vi "Keithley 2420 avg resistance.vi"() -> ()   [LabVIEW 2013]
uses:
  <instrlib>/Keithley 24XX/Public/Data/Read (Single Point).vi
  <instrlib>/Keithley 24XX/Keithley 24XX.lvlib
panel:
  in  "stop":bool
  out "Waveform Chart":cluster{sgl, sgl}(graph)
  out "avg resistance (kOhm)":sgl
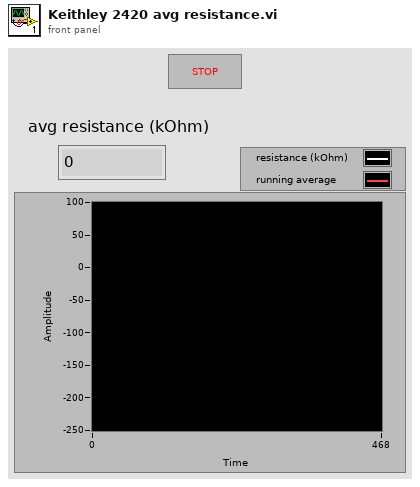
[diagram p1: front panel]
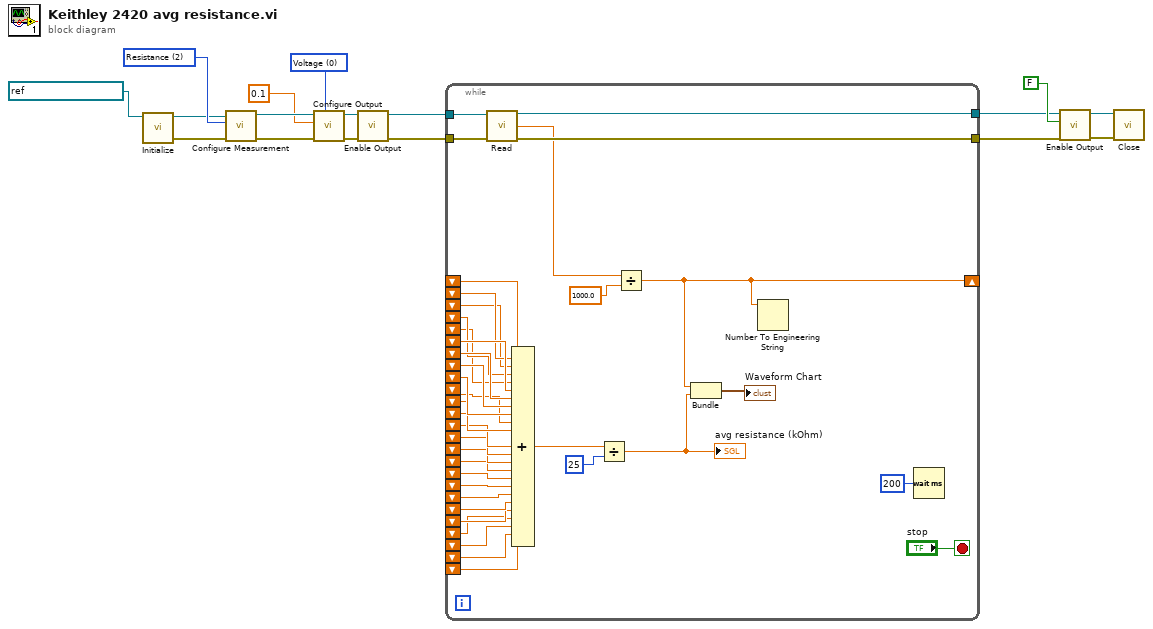
[diagram p0: block diagram]
diagram:
  w11 = u16 0 items=["Voltage", "Current"] ("Source Mode  (0: Voltage)")
  w16 = u16 2 items=["Volts", "Current", "Resistance"] ("Function (0: Volts)")
  n1 = call <instrlib>:"Initialize.vi"("VISA resource name"=refnum<visa-resource-name> "GPIB1::24::INSTR") -> ("error out"=w8:errorcluster, "VISA resource name out"=w9:refnum<visa-resource-name>)  [unwired: 9 in]
  n2 = call <instrlib>:"Configure Measurement.vi"("error in (no error)"=w8, "Function (0: Volts)"=w16, "VISA resource name"=w9) -> ("error out"=w15:errorcluster, "VISA resource name out"=w14:refnum<visa-resource-name>)  [unwired: 7 in]
  n3 = call <instrlib>:"Configure Output.vi"("Source Mode  (0: Voltage)"=w11, "error in (no error)"=w15, "Output Level (0)"=0.1, "VISA resource name"=w14) -> ("error out"=w13:errorcluster, "VISA resource name out"=w12:refnum<visa-resource-name>)  [unwired: 6 in]
  n4 = call <instrlib>:"Enable Output.vi"("error in (no error)"=w13, "VISA resource name"=w12) -> ("error out"=w1:errorcluster, "VISA resource name out"=w2:refnum<visa-resource-name>)  [unwired: 8 in]
  n5 = while {
    tunnel: [w54] -> w4
    tunnel: [w53] -> w3
    tunnel: w2 -> [w52]
    tunnel: w1 -> [w51]
    shift-right: [w24] -> _
    shift-left: _ -> [w50]
    shift-left: _ -> [w49]
    shift-left: _ -> [w48]
    shift-left: _ -> [w47]
    shift-left: _ -> [w46]
    shift-left: _ -> [w45]
    shift-left: _ -> [w44]
    shift-left: _ -> [w43]
    shift-left: _ -> [w42]
    shift-left: _ -> [w41]
    shift-left: _ -> [w35]
    shift-left: _ -> [w31]
    shift-left: _ -> [w32]
    shift-left: _ -> [w33]
    shift-left: _ -> [w34]
    shift-left: _ -> [w29]
    shift-left: _ -> [w28]
    shift-left: _ -> [w27]
    shift-left: _ -> [w26]
    shift-left: _ -> [w25]
    shift-left: _ -> [w19]
    shift-left: _ -> [w20]
    shift-left: _ -> [w21]
    shift-left: _ -> [w22]
    shift-left: _ -> [w23]
    stop <- "stop" stop-if-true
    n6 = call-poly <instrlib>:"Read.vi"("VISA resource name"=w52, "error in (no error)"=w51) -> ("VISA resource name out"=w54:refnum<visa-resource-name>, "Resistance"=w37:sgl, "error out"=w53:errorcluster)  [unwired: 7 in, 4 out]
    n7 = Compound Arithmetic op=ADD(w23, w22, w21, w20, w19, w50, w49, w48, w47, w46, w45, w44, w43, w42, w41, w35, w31, w32, w33, w34, w29, w28, w27, w26, w25) -> (w40:sgl)
    n8 = Divide(x=w40, y=25 ("# of measurements to average")) -> (x/y=w39:sgl)
    "avg resistance (kOhm)" <- w39
    n9 = Divide(x=w37, y=sgl 1000.0) -> (x/y=w24:sgl)
    n10 = Bundle(w24, w39) -> (→"Waveform Chart":cluster{sgl, sgl})  [unwired: 1 in]
    n11 = Number To Engineering String(4:w24) -> ()  [unwired: 3 in, 1 out]
    n12 = Wait (ms)(milliseconds to wait=u32 200) -> ()  [unwired: 1 out]
  }
  n13 = call <instrlib>:"Enable Output.vi"("error in (no error)"=w3, "Enable Output (T: Enable)"=FALSE, "VISA resource name"=w4) -> ("error out"=w5:errorcluster, "VISA resource name out"=w7:refnum<visa-resource-name>)  [unwired: 7 in]
  n14 = call <instrlib>:"Close.vi"("error in (no error)"=w5, "VISA resource name"=w7) -> ()  [unwired: 9 in, 1 out]
